vi "ReadMessage.vi"(7 "ConcreteMessage":refnum<class "ConcreteMessage.lvclass">) -> (3 "Message":T1 {"MessageMetadata"."AbsoluteTime" format="%<%x %.3X>T"})   [LabVIEW 2020, in "_Template.lvlib" / "MessageTemplate.lvlib" / "{{Name}}.lvlib" / "ConcreteMessage.lvclass"]
uses:
  ConcreteMessage.lvclass
  ConcreteMessage.lvclass/ConcreteMessage.ctl
  jettl/jettl/Lifetime.ctl
  jettl/jettl/jettl.lvlib
  jettl/jettl/TellOrigin.ctl
  jettl/jettl/MessageMetadata.ctl
  Message.ctl
  {{Name}}.lvlib
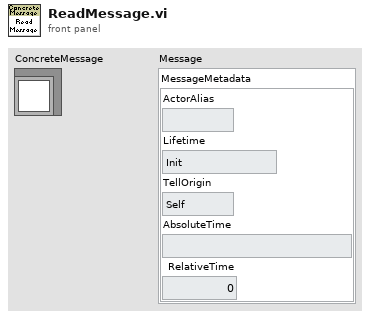
[diagram p1: front panel]
types:
  T1 = typedef "_Template.lvlib/MessageTemplate.lvlib/{{Name}}.lvlib/Message.ctl" = cluster{"MessageMetadata":T2}
  T2 = typedef "jettl.lvlib/MessageMetadata.ctl" = cluster{"ActorAlias":string, "Lifetime":T3, "TellOrigin":T4, "AbsoluteTime":timestamp, "RelativeTime":dbl}
  T3 = typedef "jettl.lvlib/Lifetime.ctl" = enum16{"Init", "Spawn", "Setup", "TeardownBeforeRunning", "Running", "StopCalled", "StoppingWithComponents", "StoppingNoComponents", "TeardownAfterRunning", "Stopped"}
  T4 = typedef "jettl.lvlib/TellOrigin.ctl" = enum16{"Self", "Mediator", "Component"}
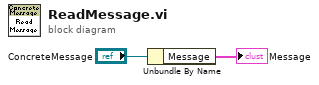
[diagram p0: block diagram]
diagram:
  n1 = Unbundle By Name("ConcreteMessage") -> ("Message"=→"Message":T1)
